vi "Code_to_run.vi"(0 "Extra command String":string, 1 "Open Front Panel":bool, 2 "Raw data option":enum16{"Save raw data", "Raw data not saved"}(ring), 3 "Current Row Comments":string, 4 "Camera Resolution":T1=1 items=["Low", "Med.", "High", "Max."], 5 "setup":T4, 7 "Remote control":bool, 9 "File":T2, 11 "Results Filename":path, 12 "Raw data file":path, 13 "Averaging time (min)":dbl=6.0 format="%.2f", 14 "Setup filename":string) -> (15 "Status":T3)   [LabVIEW 2022 SP3]
uses:
  Controls/Setup.ctl
  Multi_Run_Status.ctl
  Controls/Save_Data.ctl
  Camera Server/Camera enum/Camera resolution.ctl
  Controls/Post_Process.ctl
  Globals/Trav_pos_global.vi
  Globals/Meas_global.vi
  Globals/Constants_global.vi
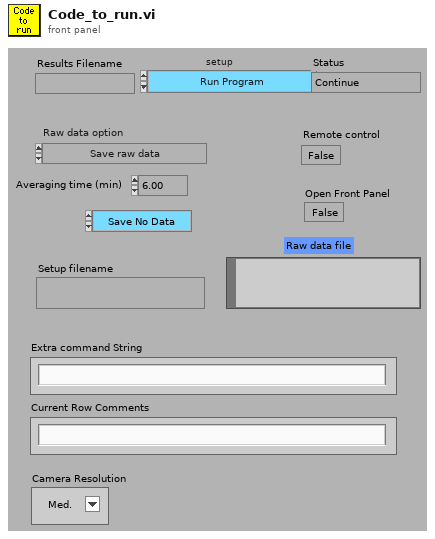
[diagram p1: front panel]
types:
  T1 = typedef "Camera resolution.ctl" = u8
  T2 = typedef "Save_Data.ctl" = enum16{"Save No Data", "Save Data"}
  T3 = typedef "Multi_Run_Status.ctl" = enum16{"Continue", "Continue with Error", "Jump to Next Point", "Jump to Next Row", "Jump To Fall Back", "Terminate Run"}
  T4 = typedef "Setup.ctl" = enum16{"Run Program", "Show Setup", "Save Current Setup", "Setup Front Panel"}
  T5 = typedef "Post_Process.ctl" = enum16{"Take New Data", "Post Process Raw Data File"}
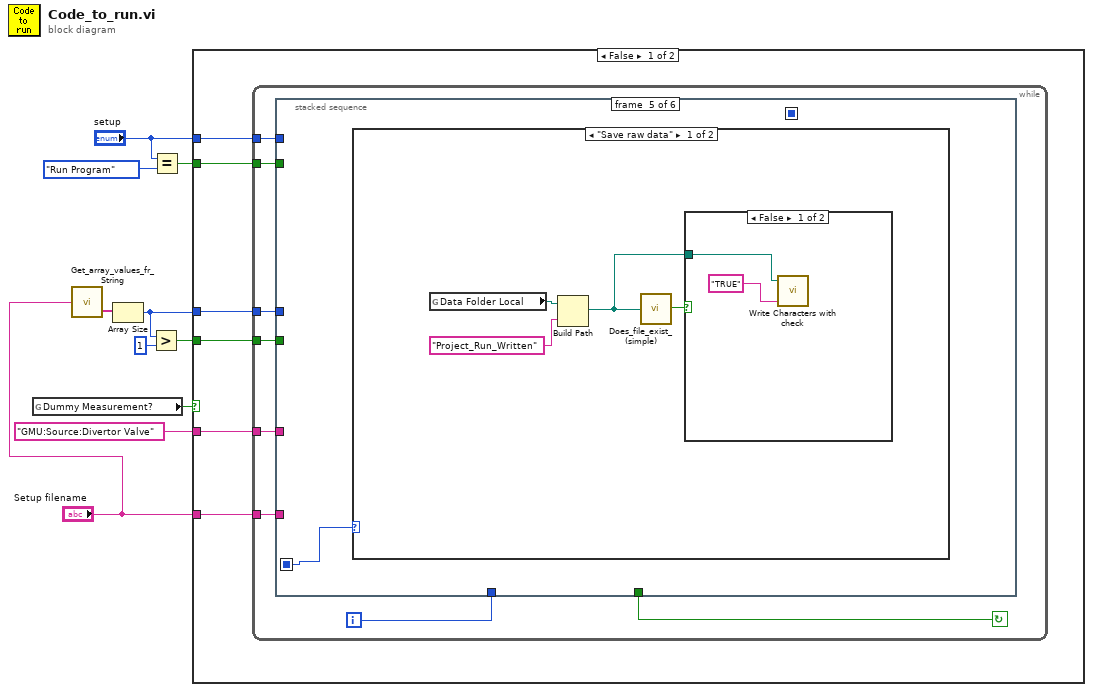
[diagram p0: block diagram]
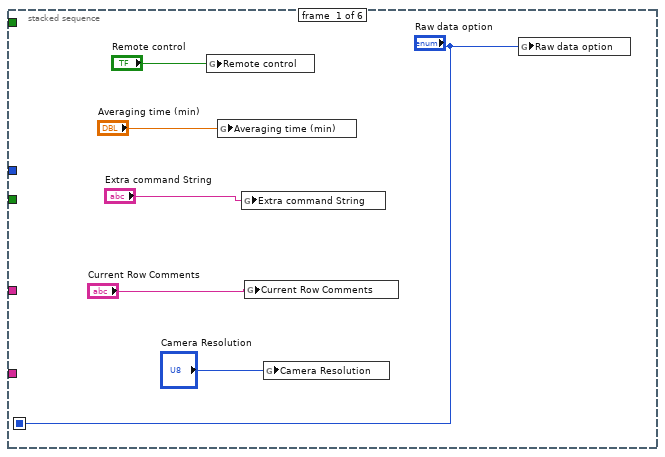
[diagram p2: hidden frame]
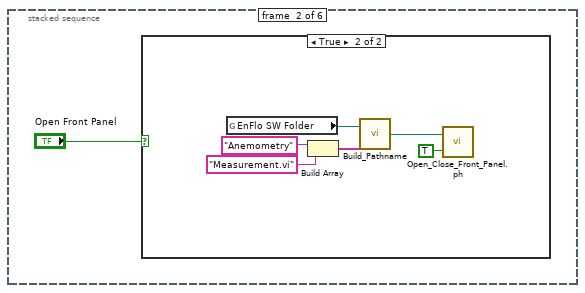
[diagram p3: hidden frame]
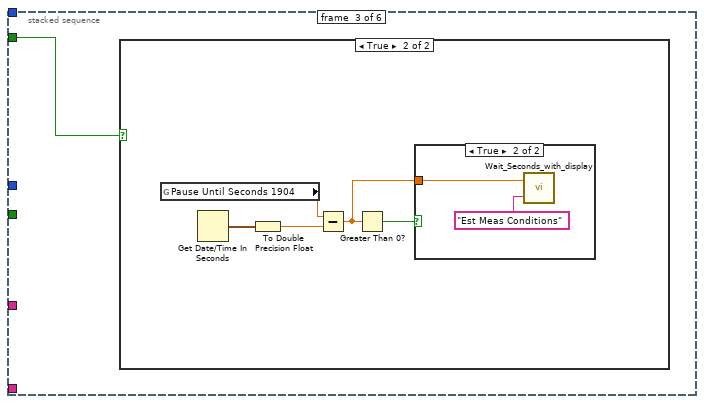
[diagram p5: hidden frame]
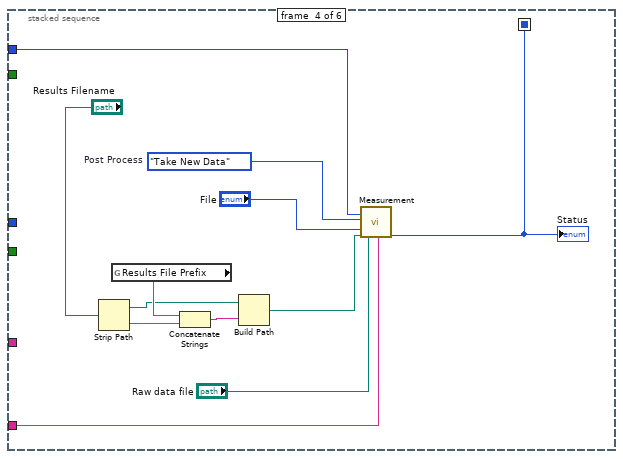
[diagram p8: hidden frame]
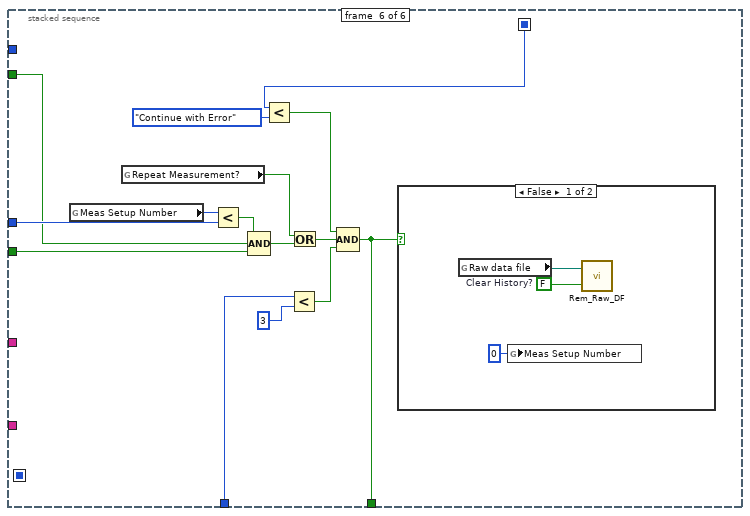
[diagram p11: hidden frame]
diagram:
  n1 = global read "Trav_pos_global.vi" "Dummy Measurement?"() -> (w10:bool)
  n2 = call "Get_array_values_fr_String.vi"("String Value"="Setup filename") -> ("String array"=w9:string[])  [unwired: 1 out]
  n3 = Array Size(array=w9) -> (size(s)=w7:i32)
  n4 = Greater?(x=w7, y=1) -> (0:w6:bool)
  n5 = Equal?(x="setup", y=Setup."Run Program" ("setup")) -> (x = y?=w3:bool)
  n6 = case shown="False" w10 {
    tunnel: w7 -> [w16 _]
    tunnel: w6 -> [w15 _]
    tunnel: "setup" -> [w14 _]
    tunnel: w3 -> [w13 _]
    tunnel: "GMU:Source:Divertor Valve" -> [w12 _]
    tunnel: "Setup filename" -> [w11 _]
    frame False {
      n7 = while {
        tunnel: w16 -> [w23]
        tunnel: w15 -> [w22]
        tunnel: w14 -> [w21]
        tunnel: w13 -> [w20]
        tunnel: w12 -> [w19]
        tunnel: w11 -> [w18]
        i -> [w17]
        stop <- w24 continue-if-true
        n8 = stacked-sequence {
          seq-local: [_ _ _ w54 _ _] -> [_ _ _ _ _ w78]
          seq-local: ["Raw data option" _ _ _ _ _] -> [_ _ _ _ w58 _]
          tunnel: [_ _ _ _ _ w71] -> w24
          tunnel: w23 -> [_ _ _ _ _ w76]
          tunnel: w22 -> [_ _ _ _ _ w65]
          tunnel: w21 -> [_ _ _ w53 _ _]
          tunnel: w20 -> [_ _ w38 _ _ w66]
          tunnel: w19 -> [_ _ _ _ _ _]
          tunnel: w18 -> [_ _ _ w52 _ _]
          tunnel: w17 -> [_ _ _ _ _ w70]
          frame #0 {
            n9 = global write "Meas_global.vi" "Remote control"("Remote control") -> ()
            n10 = global write "Meas_global.vi" "Averaging time (min)"("Averaging time (min)") -> ()
            n11 = global write "Meas_global.vi" "Extra command String"("Extra command String") -> ()
            n12 = global write "Meas_global.vi" "Current Row Comments"("Current Row Comments") -> ()
            n13 = global write "Meas_global.vi" "Camera Resolution"("Camera Resolution") -> ()
            n14 = global write "Meas_global.vi" "Raw data option"("Raw data option") -> ()
          }
          frame #1 {
            n15 = case shown="True" "Open Front Panel" {
              frame False {
              }
              frame True {
                n16 = global read "Constants_global.vi" "EnFlo SW Folder"() -> (w34:path)
                n17 = Build Array("Anemometry", "Measurement.vi") -> (w35:string[])
                n18 = call "Build_Pathname.vi"("PathElements"=w35, "PathnameIn"=w34) -> ("AppendedPath"=w33:path)
                n19 = call "Open_Close_Front_Panel.ph.vi"("openWindow (T)"=TRUE ("Front Panel Window:Open"), "VI path"=w33) -> ()  [unwired: 1 in, 1 out]
              }
            }
          }
          frame #2 {
            n20 = case shown="True" w38 {
              frame False {
              }
              frame True {
                n21 = global read "Trav_pos_global.vi" "Pause Until Seconds 1904"() -> (w43:dbl)
                n22 = Get Date/Time In Seconds() -> (seconds since 1Jan1904=w42:timestamp)
                n23 = To Double Precision Float(number=w42) -> (double precision float=w41:dbl)
                n24 = Subtract(x=w43, y=w41) -> (x-y=w39:dbl)
                n25 = Greater Than 0?(x=w39) -> (x > 0?=w40:bool)
                n26 = case shown="True" w40 {
                  tunnel: w39 -> [_ w44]
                  frame False {
                  }
                  frame True {
                    n27 = call "Wait_Seconds_with_display.vi"("Message"="Est Meas Conditions", "Seconds to wait"=w44) -> ()  [unwired: 2 out]
                  }
                }
              }
            }
          }
          frame #3 {
            w55 = Post_Process."Take New Data"  # Post Process
            n28 = Strip Path(path="Results Filename") -> (stripped path=w47:path, name=w50:string)
            n29 = global read "Trav_pos_global.vi" "Results File Prefix"() -> (w49:string)
            n30 = Concatenate Strings(w49, w50) -> (w48:string)
            n31 = Build Path(base path=w47, name or relative path=w48) -> (appended path=w46:path)
            n32 = call "Measurement.vi"("setup"=w53, "Post Process"=w55, "File"="File", "Results file"=w46, "Raw data file"="Raw data file", "Setup filename"=w52) -> ("Status Out"=w54:T3)  [unwired: 13 out]
            "Status" <- w54
          }
          frame #4 {
            n33 = case shown="\"Save raw data\"" w58 {
              frame "Save raw data" {
                n34 = global read "Constants_global.vi" "Data Folder Local"() -> (w61:path)
                n35 = Build Path(base path=w61, name or relative path="Project_Run_Written") -> (appended path=w59:path)
                n36 = call "Does_file_exist_(simple).vi"("Pathname"=w59) -> ("exists?"=w60:bool)
                n37 = case shown="False" w60 {
                  tunnel: w59 -> [w64 _]
                  frame False {
                    n38 = call "Write Characters with check.vi"("String to Write"="TRUE" ("text"), "file (use dialog)"=w64) -> ()  [unwired: 2 in, 1 out]
                  }
                  frame True {
                  }
                }
              }
              frame "Raw data not saved" {
              }
            }
          }
          frame #5 {
            n39 = global read "Trav_pos_global.vi" "Meas Setup Number"() -> (w77:i32)
            n40 = global read "Meas_global.vi" "Repeat Measurement?"() -> (w74:bool)
            n41 = Less?(x=w77, y=w76) -> (x < y?=w67:bool)
            n42 = Compound Arithmetic op=AND(w67, w66, w65) -> (w75:bool)
            n43 = Less?(x=w78, y=Multi_Run_Status."Continue with Error" ("Status Out")) -> (x < y?=w72:bool)
            n44 = Less?(x=w70, y=3) -> (x < y?=w68:bool)
            n45 = Or(x=w74, y=w75) -> (x .or. y?=w73:bool)
            n46 = Compound Arithmetic op=AND(w72, w73, w68) -> (w71:bool)
            n47 = case shown="False" w71 {
              frame False {
                w81 = FALSE  # Clear History?
                n48 = global read "Meas_global.vi" "Raw data file"() -> (w82:path)
                n49 = global write "Trav_pos_global.vi" "Meas Setup Number"(0 ("Meas Setup Number")) -> ()
                n50 = call "Rem_Raw_DF.vi"("Clear History?"=w81, "Filename to Remember"=w82) -> ()  [unwired: 1 out]
              }
              frame True {
              }
            }
          }
        }
      }
    }
    frame True {
    }
  }
